vi "ReadAttributesTest.vi"() -> ()   [LabVIEW 2013, in "examples.lvlib"]
uses:
  examples.lvlib
  vis/lv-2013/tango_vi.llb/avToShortImage.vi
  vis/lv-2013/tango_vi.llb/avToLongSpectrum.vi
  vis/lv-2013/tango_vi.llb/avToDoubleScalar.vi
  vis/lv-2013/tango_vi.llb/avToStringScalarAv.vi
  vis/lv-2013/tango_vi.llb/tango.lvlib
panel:
  out "timestamp":string="sam. 28/01/06 19:14:33,51"
  out "?":string
  out "attribute name":string="string_scalar"
  out "quality":string="VALID"
  out "?":i16[][](graph)
  out "value":dbl(graph)
  out "?":i32[](graph)
  out "success":bool=TRUE
  in  "<TangoTest> device name":string="sys/tg_test/1"
  in  "Attribute names":string[](array[string])=["double_scalar", "long_spectrum_ro", "short_image_ro", "string_scalar"]
  # "TANGO  Binding for LabVIEW - ReadAttributes example"
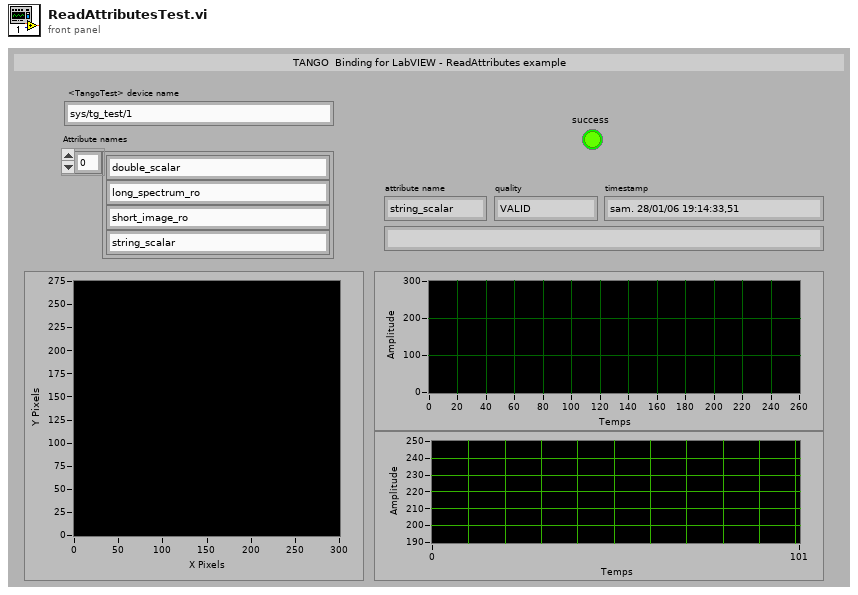
[diagram p1: front panel]
types:
  T1 = cluster{"device name":string, "attribute name":string, "quality value":i16, "quality string":string, "timestamp":dbl, "dim. x":i32, "dim. y":i32, "value":u8[], "error code":i32, "error stack":string[], "data type":u16}[]
  T2 = cluster{"device name":string, "attribute name":string, "quality value":i16, "quality string":string, "timestamp":dbl, "dim. x":i32, "dim. y":i32, "value":u8[], "error code":i32, "error stack":string[], "data type":u16}
  T3 = cluster{"device name":string, "attribute name":string, "quality value":i16, "quality string":string, "timestamp":dbl, "dim. x":i32, "dim. y":i32, "value_out":string, "setpoint":string, "error code":i32, "error stack":string[], "data type":u16}
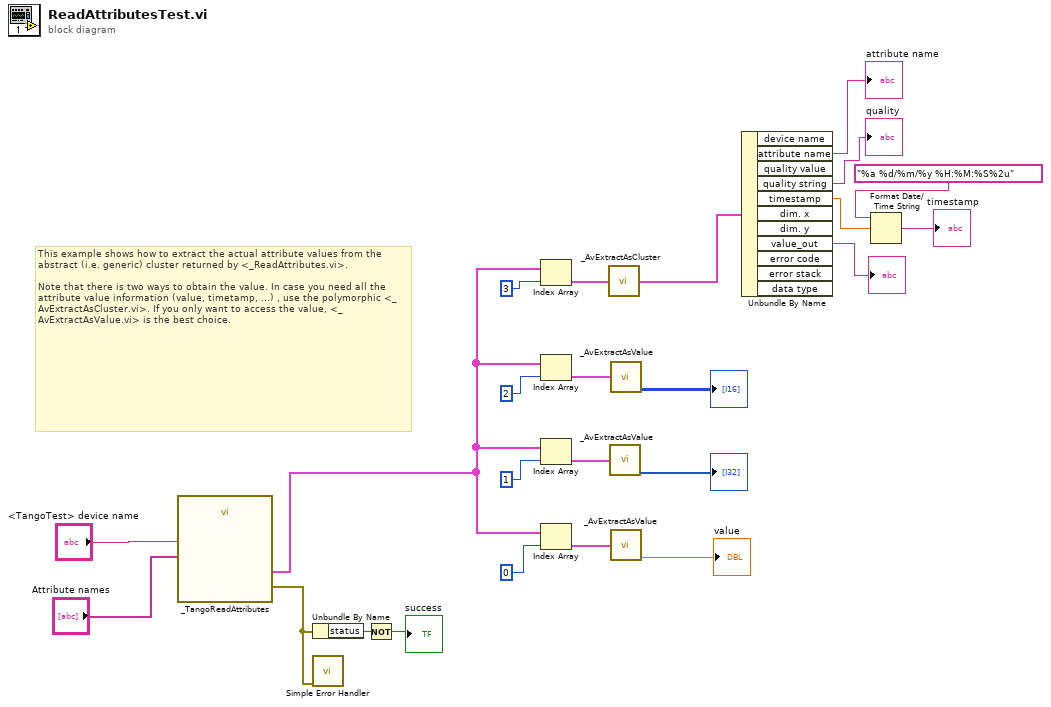
[diagram p0: block diagram]
diagram:
  # "This example shows how to extract the actual attribute values from the abstract (i.e. generic) cluster returned by <_ReadAttributes.vi>. \n\nNote that there is two ways to obtain the value. In case you need all the attribute value information (value, timetamp, ...) , use the polymorphic <_AvExtractAsCluster.vi>. If you only want to access the value, <_AvExtractAsValue.vi> is the best choice."
  n1 = call "_TangoReadAttributes.vi"("attribute names"="Attribute names", "device name"="<TangoTest> device name") -> ("error out"=w2:errorcluster, "attribute values"=w24:T1)  [unwired: 1 in]
  n2 = Unbundle By Name(w2) -> ("status"=w3:bool)
  n3 = call <vilib>:"Simple Error Handler.vi"("error in (no error)"=w2) -> ()  [unwired: 4 in, 5 out]
  n4 = Not(x=w3) -> (.not. x?=→"success":bool)
  n5 = Index Array(array=w24, index=3 ("indice")) -> (element=w8:T2)
  n6 = Index Array(array=w24, index=2 ("indice")) -> (element=w7:T2)
  n7 = Index Array(array=w24, index=1 ("indice")) -> (element=w6:T2)
  n8 = Index Array(array=w24, index=0 ("indice")) -> (element=w5:T2)
  n9 = call-poly "_AvExtractAsCluster.vi"("attribute value"=w8) -> ("av"=w15:T3)
  n10 = call-poly "_AvExtractAsValue.vi"("attribute value"=w6) -> ("value"=→"?":i32[])  [unwired: 4 out]
  n11 = call-poly "_AvExtractAsValue.vi"("attribute value"=w7) -> ("value"=→"?":i16[][])  [unwired: 4 out]
  n12 = call-poly "_AvExtractAsValue.vi"("attribute value"=w5) -> ("value"=→"value":dbl)  [unwired: 4 out]
  n13 = Unbundle By Name(w15) -> ("attribute name"=→"attribute name":string, "quality string"=→"quality":string, "timestamp"=w14:dbl, "value_out"=→"?":string)  [unwired: 7 out]
  n14 = Format Date/Time String(time format string (%c)="%a %d/%m/%y %H:%M:%S%2u" ("chaîne de format de l'heure (%c)"), seconds (now)=w14) -> (date/time string=→"timestamp":string)  [unwired: 1 in]
